vi "handle list.vi"(0 "operation":T1(ring), 3 "index":i8, 4 "input entry":i32, 6 "colume":i32, 7 "new element/subarray":string, 8 "add to list":dbl[](array[numeric]), 9 "channel":i8) -> (12 "exp.list":string[][](array[string]), 13 "subarray":string[](array[string]), 16 "output entry":i32, 19 "done":bool)   [LabVIEW 2023]
uses:
  <vilib>/Utility/file.llb/Read Delimited Spreadsheet (string).vi
  <vilib>/Utility/file.llb/Write Delimited Spreadsheet (string).vi
  <vilib>/Utility/file.llb/Write Delimited Spreadsheet (DBL).vi
  Shared variables/exp.list.vi
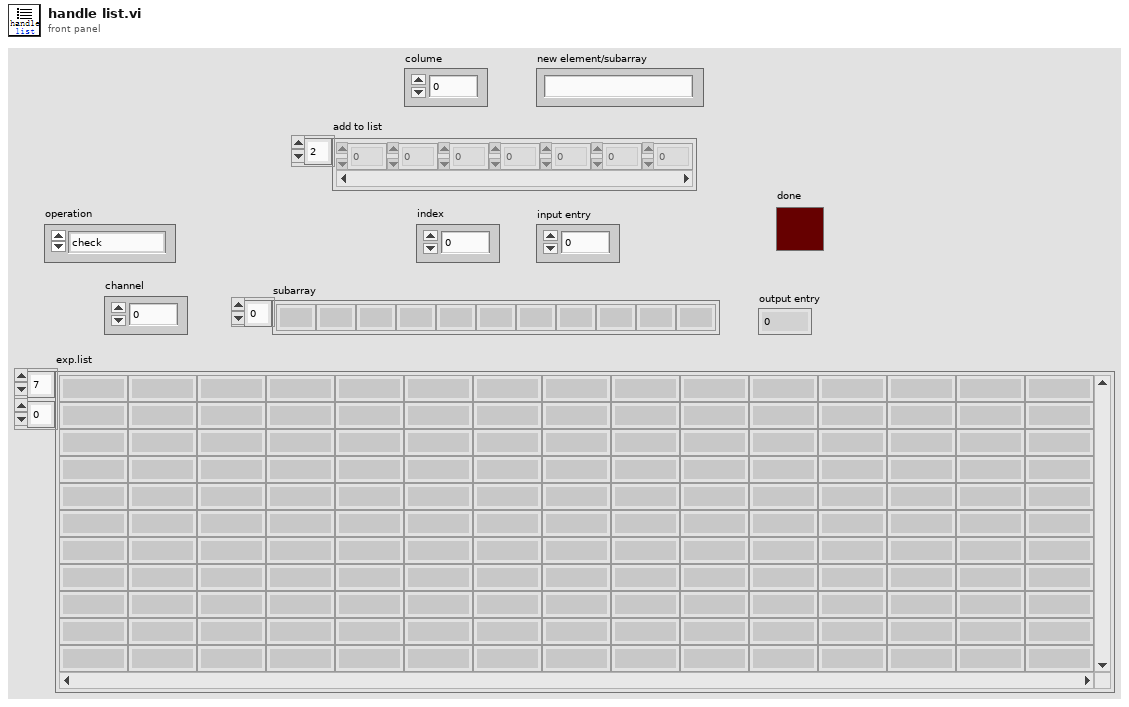
[diagram p1: front panel]
types:
  T1 = enum16{"check", "scan", "index", "read", "add", "write"}
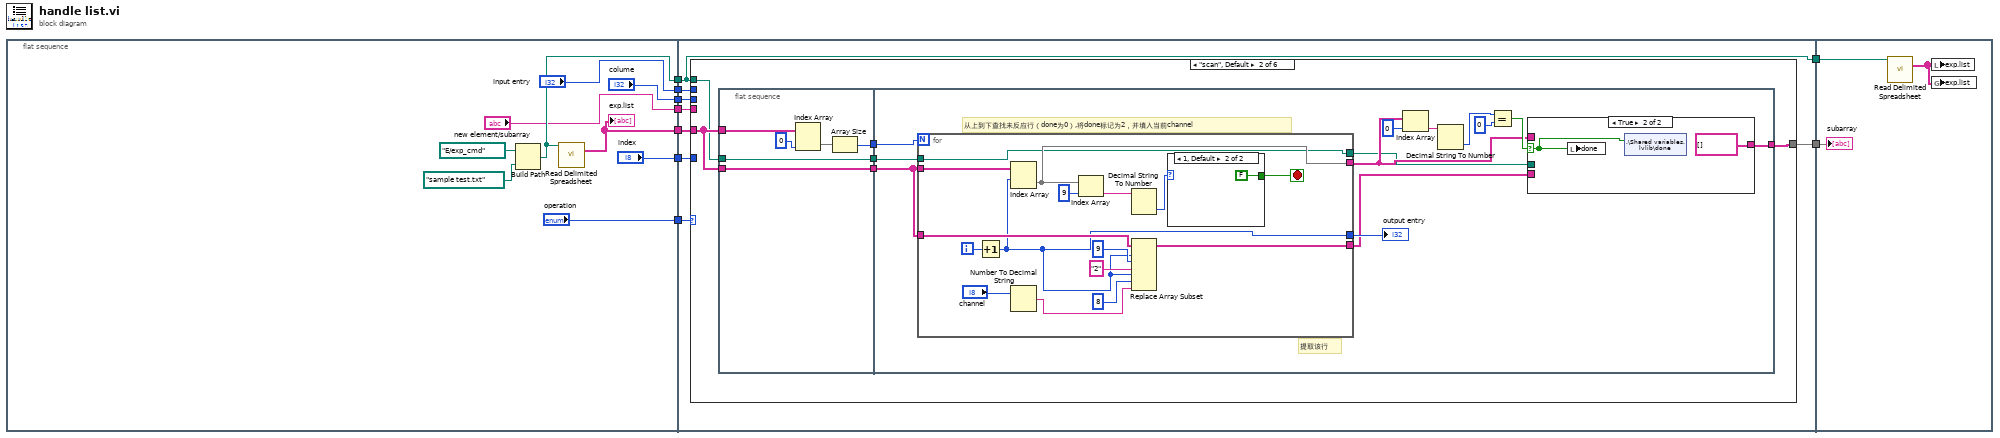
[diagram p0: block diagram]
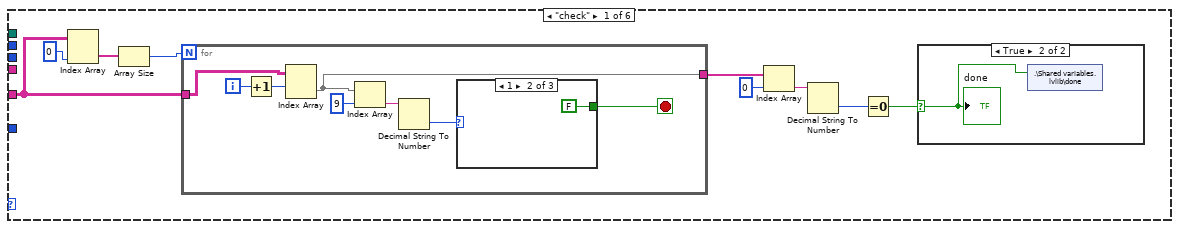
[diagram p2: hidden frame]
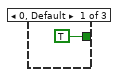
[diagram p4: hidden frame]
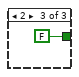
[diagram p5: hidden frame]
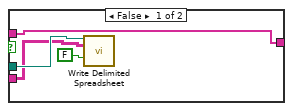
[diagram p6: hidden frame]
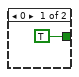
[diagram p7: hidden frame]
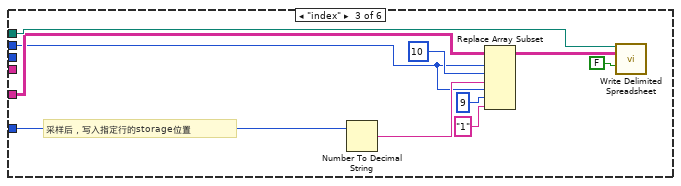
[diagram p8: hidden frame]
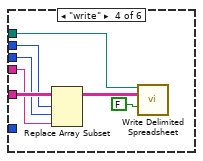
[diagram p9: hidden frame]
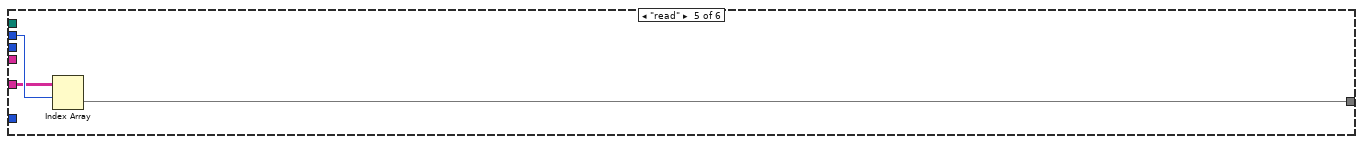
[diagram p10: hidden frame]
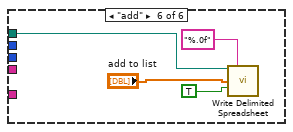
[diagram p11: hidden frame]
diagram:
  n1 = flat-sequence {
    tunnel: [w16] -> w9
    tunnel: [w15] -> w8
    tunnel: ["operation"] -> w7
    tunnel: ["input entry"] -> w5
    tunnel: ["index"] -> w4
    tunnel: ["colume"] -> w2
    tunnel: ["new element/subarray"] -> w1
    tunnel: w9 -> [w25]
    tunnel: w8 -> [w24]
    tunnel: w7 -> [w26]
    tunnel: [w24] -> w6
    tunnel: w5 -> [w23]
    tunnel: w4 -> [w22]
    tunnel: [w21] -> w3
    tunnel: w2 -> [w20]
    tunnel: w1 -> [w19]
    tunnel: w6 -> [w122]
    tunnel: w3 -> [w121]
    frame #0 {
      n2 = Build Path(base path=path "E:/exp_cmd", name or relative path=path "sample test.txt") -> (appended path=w15:path)
      n3 = call-poly <vilib>:"Read Delimited Spreadsheet.vi"("file path (dialog if empty)"=w15) -> ("all rows"=w16:string[][])  [unwired: 9 in, 5 out]
      "exp.list" <- w16
    }
    frame #1 {
      n4 = case shown="\"scan\", Default" w26 {
        tunnel: w25 -> [w33 w50 w101 w110 w115 _]
        tunnel: w24 -> [_ w49 w102 w111 _ w117]
        tunnel: w23 -> [_ _ w98 w109 w116 _]
        tunnel: w22 -> [_ _ w97 _ _ _]
        tunnel: [_ w48 _ _ w114 _] -> w21
        tunnel: w20 -> [_ _ _ w108 _ _]
        tunnel: w19 -> [_ _ _ w107 _ _]
        frame "check" {
          n5 = Index Array(array=w33, index (col)=0 ("disabled index (col)")) -> (element=w35:string[])  [unwired: 1 in]
          n6 = Array Size(array=w35) -> (size(s)=w27:i32)
          n7 = for {
            N: w27 -> [_]
            tunnel: w33 -> [w44]
            tunnel: [w37] -> w31
            i -> [w43]
            stop <- w38 stop-if-true
            n8 = Increment(x=w43) -> (x+1=w42:i32)
            n9 = Index Array(array=w44, index (row)=w42) -> (element=w37:string[])  [unwired: 1 in]
            n10 = Index Array(array=w37, index=9) -> (element=w40:string)
            n11 = Decimal String To Number(string=w40) -> (number=w39:i32)  [unwired: 2 in, 1 out]
            n12 = case shown="1" w39 {
              tunnel: [TRUE FALSE FALSE] -> w38
              frame 0, Default {
              }
              frame 1 {
              }
              frame 2 {
              }
            }
          }
          n13 = Index Array(array=w31, index=0) -> (element=w30:string)
          n14 = Decimal String To Number(string=w30) -> (number=w29:i32)  [unwired: 2 in, 1 out]
          n15 = Equal To 0?(x=w29) -> (x = 0?=w28:bool)
          n16 = case shown="True" w28 {
            selector: w28 -> [_ w36]
            frame False {
            }
            frame True {
              n17 = shared-variable ".\\Shared variables.lvlib\\done"(w36) -> ()  [unwired: 1 in, 1 out]
              "done" <- w36
            }
          }
        }
        frame "scan", Default {
          n18 = flat-sequence {
            tunnel: [w56] -> w53
            tunnel: [w54] -> w52
            tunnel: [w55] -> w51
            tunnel: w50 -> [w57]
            tunnel: w50 -> [w56]
            tunnel: w49 -> [w55]
            tunnel: w53 -> [w72]
            tunnel: w52 -> [w66]
            tunnel: w51 -> [w71]
            tunnel: [w64] -> w48
            frame #0 {
              n19 = Index Array(array=w57, index (col)=0 ("disabled index (col)")) -> (element=w59:string[])  [unwired: 1 in]
              n20 = Array Size(array=w59) -> (size(s)=w54:i32)
            }
            frame #1 {
              # "提取该行"
              # "从上到下查找未反应行（done为0）,将done标记为2，并填入当前channel"
              n21 = for {
                N: w66 -> [_]
                tunnel: w72 -> [w92]
                tunnel: w71 -> [w79]
                tunnel: w72 -> [w91]
                tunnel: [w86] -> w63
                tunnel: [w82] -> w70
                tunnel: [w79] -> w61
                tunnel: [w80] -> w60
                i -> [w88]
                stop <- w87 stop-if-true
                n22 = Increment(x=w88) -> (x+1=w82:i32)
                n23 = Index Array(array=w92, index (row)=w82) -> (element=w86:string[])  [unwired: 1 in]
                n24 = Number To Decimal String(number="channel") -> (decimal integer string=w81:string)  [unwired: 1 in]
                n25 = Index Array(array=w86, index=9) -> (element=w94:string)
                n26 = Decimal String To Number(string=w94) -> (number=w85:i32)  [unwired: 2 in, 1 out]
                n27 = Replace Array Subset(array=w91, new element #1="2" ("new element/subarray"), index (row) #1=w82, index (col) #1=9 ("disabled index (col)"), new element #2=w81, index (row) #2=w82, index (col) #2=8 ("disabled index (col)")) -> (w80:string[][])
                n28 = case shown="1, Default" w85 {
                  tunnel: [TRUE FALSE] -> w87
                  frame 0 {
                  }
                  frame 1, Default {
                  }
                }
              }
              "output entry" <- w70
              n29 = Index Array(array=w63, index=0) -> (element=w68:string)
              n30 = Decimal String To Number(string=w68) -> (number=w67:i32)  [unwired: 2 in, 1 out]
              n31 = Equal?(x=w67, y=0) -> (x = y?=w65:bool)
              n32 = case shown="True" w65 {
                selector: w65 -> [_ w77]
                tunnel: [w76 string[] [] ("all rows")] -> w64
                tunnel: w63 -> [w76 _]
                tunnel: w61 -> [w75 _]
                tunnel: w60 -> [w74 _]
                frame False {
                  n33 = call-poly <vilib>:"Write Delimited Spreadsheet.vi"("file path (dialog if empty)"=w75, "2D data"=w74, "append to file? (new file:F)"=FALSE) -> ()  [unwired: 11 in, 2 out]
                }
                frame True {
                  n34 = local write "done"(w77) -> ()
                  n35 = shared-variable ".\\Shared variables.lvlib\\done"(w77) -> ()  [unwired: 1 in, 1 out]
                }
              }
            }
          }
        }
        frame "index" {
          # "采样后，写入指定行的storage位置"
          n36 = Number To Decimal String(number=w97) -> (decimal integer string=w103:string)  [unwired: 1 in]
          n37 = Replace Array Subset(array=w101, new element #1=w103, index (row) #1=w98, index (col) #1=10 ("disabled index (col)"), new element #2="1" ("new element/subarray"), index (row) #2=w98, index (col) #2=9 ("disabled index (col)")) -> (w105:string[][])
          n38 = call-poly <vilib>:"Write Delimited Spreadsheet.vi"("file path (dialog if empty)"=w102, "2D data"=w105, "append to file? (new file:F)"=FALSE) -> ()  [unwired: 11 in, 2 out]
        }
        frame "write" {
          n39 = Replace Array Subset(array=w110, new element=w107, index (row)=w109, index (col)=w108) -> (w113:string[][])
          n40 = call-poly <vilib>:"Write Delimited Spreadsheet.vi"("file path (dialog if empty)"=w111, "2D data"=w113, "append to file? (new file:F)"=FALSE) -> ()  [unwired: 11 in, 2 out]
        }
        frame "read" {
          n41 = Index Array(array=w115, index (row)=w116) -> (element=w114:string[])  [unwired: 1 in]
        }
        frame "add" {
          n42 = call-poly <vilib>:"Write Delimited Spreadsheet.vi"("file path (dialog if empty)"=w117, "format (%.3f)"="%.0f", "1D data"="add to list", "append to file? (new file:F)"=TRUE) -> ()  [unwired: 10 in, 2 out]
        }
      }
    }
    frame #2 {
      n43 = call-poly <vilib>:"Read Delimited Spreadsheet.vi"("file path (dialog if empty)"=w122) -> ("all rows"=w123:string[][])  [unwired: 9 in, 5 out]
      n44 = local write "exp.list"(w123) -> ()
      n45 = global write "exp.list.vi" "exp.list"(w123) -> ()
      "subarray" <- w121
    }
  }
